vi "AnalysisObjectArray_write_and_unlock.vi"(8 "error in (no error)":errorcluster, 11 "AnalysisObjects":refnum<class "Analysis.lvclass">[](array[class])) -> (0 "error out":errorcluster)   [LabVIEW 2017]
doc: "the VI writes and unlocks the AnalysisObjectsArray using a Queue"
uses:
  Classes/Analysis/Analysis.lvclass
  global variables.vi
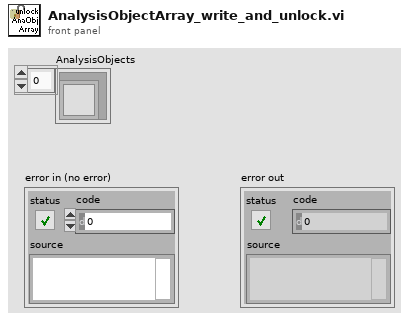
[diagram p1: front panel]
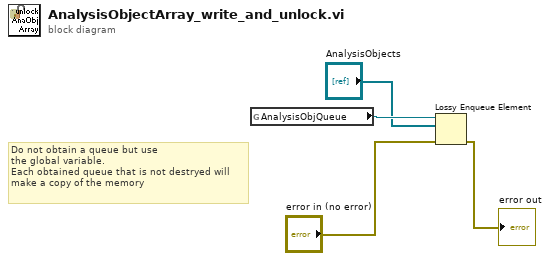
[diagram p0: block diagram]
diagram:
  # "Do not obtain a queue but use\nthe global variable.\nEach obtained queue that is not destryed will\nmake a copy of the memory"
  n1 = global read "global variables.vi" "AnalysisObjQueue"() -> (w3:refnum<queue>)
  n2 = Lossy Enqueue Element(queue=w3, element="AnalysisObjects", error in (no error)="error in (no error)") -> (error out=→"error out":errorcluster)  [unwired: 3 out]
